vi "Kickdown.vi"(11 "Cluster":T1) -> (3 "Shift?":bool)   [LabVIEW 2013]
uses:
  Drive Train Metrics.ctl
  CmdFlag.ctl
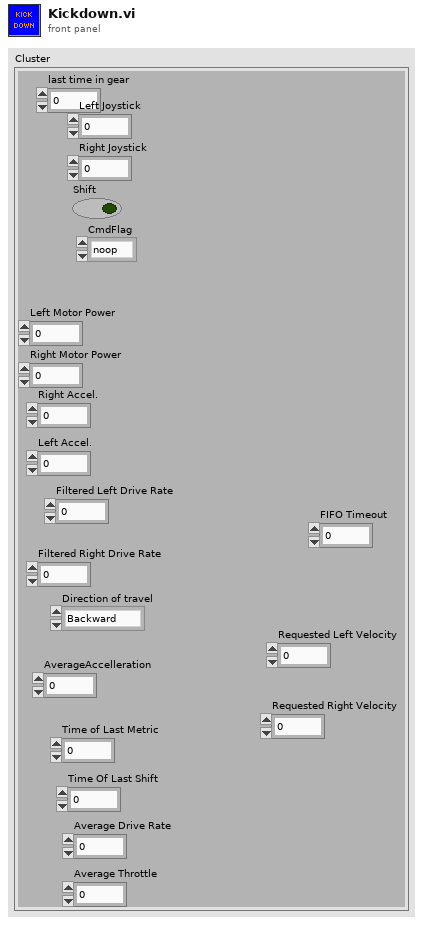
[diagram p1: front panel]
types:
  T1 = typedef "Drive Train Metrics.ctl" = cluster{"last time in gear":u32, "Shift":bool, "Right Joystick":dbl, "Left Joystick":dbl, "CmdFlag":T2, "Right Motor Power":dbl, "Left Motor Power":dbl, "Right Accel.":dbl, "Left Accel.":dbl, "Filtered Left Drive Rate":dbl, "Filtered Right Drive Rate":dbl, "Direction of travel":enum16{"Backward", "Forward", "Spin"}, "AverageAccelleration":dbl, "Time of Last Metric":u32, "Time Of Last Shift":dbl, "Average Drive Rate":dbl, "Average Throttle":dbl, "FIFO Timeout":i32, "Requested Left Velocity":dbl, "Requested Right Velocity":dbl}
  T2 = typedef "CmdFlag.ctl" = enum16{"noop", "suspend", "resume"}
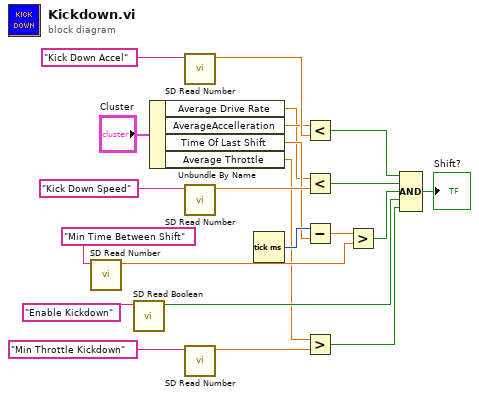
[diagram p0: block diagram]
diagram:
  n1 = call <vilib>:"SD Read Number.vi"("Name"="Min Time Between Shift") -> ("Numeric"=w13:dbl)  [unwired: 8 in, 2 out]
  n2 = call <vilib>:"SD Read Boolean.vi"("Name"="Enable Kickdown") -> ("Boolean"=w5:bool)  [unwired: 8 in, 2 out]
  n3 = Unbundle By Name("Cluster") -> ("Average Drive Rate"=w11:dbl, "AverageAccelleration"=w17:dbl, "Time Of Last Shift"=w15:dbl, "Average Throttle"=w4:dbl)
  n4 = call <vilib>:"SD Read Number.vi"("Name"="Kick Down Accel") -> ("Numeric"=w21:dbl)  [unwired: 8 in, 2 out]
  n5 = call <vilib>:"SD Read Number.vi"("Name"="Kick Down Speed") -> ("Numeric"=w22:dbl)  [unwired: 8 in, 2 out]
  n6 = call <vilib>:"SD Read Number.vi"("Name"="Min Throttle Kickdown") -> ("Numeric"=w3:dbl)  [unwired: 8 in, 2 out]
  n7 = Tick Count (ms)() -> (millisecond timer value=w16:u32)
  n8 = Less?(x=w17, y=w21) -> (x < y?=w9:bool)
  n9 = Less?(x=w11, y=w22) -> (x < y?=w10:bool)
  n10 = Subtract(x=w16, y=w15) -> (x-y=w14:dbl)
  n11 = Greater?(x=w4, y=w3) -> (0:w1:bool)
  n12 = Greater?(x=w14, y=w13) -> (0:w8:bool)
  n13 = Compound Arithmetic op=AND(w9, w10, w8, w5, w1) -> (→"Shift?":bool)
